vi "ExSpectGetSlitInfo.vi"() -> ()   [LabVIEW 2010]
panel:
  out "Speed":dbl format="%.2f"
  out "Position":dbl format="%.2f"
  in  "Slit Number":i16=1 min=1 max=4 step=1
  out "error out":errorcluster
  in  "error in (no error)":errorcluster
  # "ExSpectGetSlitInfo.vi\n(Normal Spectrograph via USB/COM port)\nThis VI will read the current position and speed of the selected slit."
  # "um"
  # "1 = Front Entrance\n 2 = Side Entrance\n 3 = Front Exit\n 4 = Side Exit"
  # "NOTES:\nA properly configured spectometer .ini must be present in the LabVIEW folder for spectrograph operation.\n\nConsult the Toolkit documentation for more information on how to configure this file."
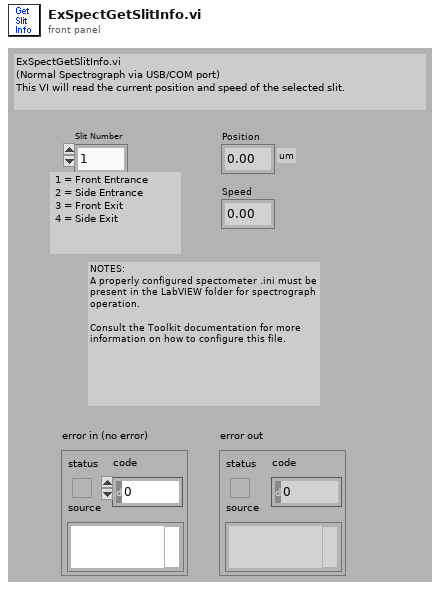
[diagram p1: front panel]
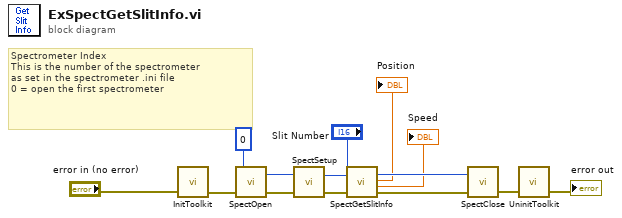
[diagram p0: block diagram]
diagram:
  # "Spectrometer Index\nThis is the number of the spectrometer\nas set in the spectrometer .ini file\n0 = open the first spectrometer"
  n1 = call <userlib>:"InitToolkit.vi"("error in"="error in (no error)") -> ("error out"=w13:errorcluster)
  n2 = call <userlib>:"SpectOpen.vi"("error in"=w13, "Spectrometer ID"=0) -> ("error out"=w12:errorcluster, "Spectrometer Handle"=w6:u32)  [unwired: 1 in]
  n3 = call <userlib>:"SpectSetup.vi"("error in"=w12, "Spectrometer Handle"=w6) -> ("error out"=w11:errorcluster, "Spectrometer Handle"=w5:u32)
  n4 = call <userlib>:"SpectGetSlitInfo.vi"("Spectrometer Handle"=w5, "Slit"="Slit Number", "error in"=w11) -> ("Spectrometer Handle"=w4:u32, "Position"=→"Position":dbl, "Speed"=→"Speed":dbl, "error out"=w10:errorcluster)
  n5 = call <userlib>:"SpectClose.vi"("error in"=w10, "Spectrometer Handle"=w4) -> ("error out"=w9:errorcluster)
  n6 = call <userlib>:"UninitToolkit.vi"("error in"=w9) -> ("error out"=→"error out":errorcluster)
